vi "FPGA.vi"() -> ()   [LabVIEW 2013]
uses:
  <vilib>/rvi/Emulation/niFpgaSctlEmulationGetInTimedLoop.vi
  <vilib>/rvi/Emulation/niFpgaEmulationReportErrorSimple.vi
  <vilib>/rvi/eio/common/nirviEmuTemplateMethod_errors.vi
  <vilib>/rvi/Emulation/niFpgaGetClockAttributes.vi
  <vilib>/rvi/Emulation/niFpgaCriticalErrorInLSC.vi
  <vilib>/eio/EIONode/EIONode.xnode
panel:
  out "Test1":bool
  out "Test2":bool
  out "Test3":bool
  out "Test4":bool
  out "GbxEnc1":i64
  out "GbxEnc2":i64
  out "GbxEnc3":i64
  out "GbxEnc4":i64
  in  "FPGA LED":bool
  out "Chasis Temp":i16
  in  "Motor5":u16 max=512 step=1
  in  "Motor6":u16 max=512 step=1
  in  "Motor7":u16 max=512 step=1
  in  "Motor8":u16 max=512 step=1
  in  "Motor9":u16 max=512 step=1
  in  "Motor10":u16 max=512 step=1
  in  "Motor11":u16 max=512 step=1
  in  "Motor12":u16 max=512 step=1
  in  "Motor1":u16 max=512 step=1
  in  "Motor2":u16 max=512 step=1
  in  "Motor3":u16 max=512 step=1
  in  "Motor4":u16 max=512 step=1
  in  "Halt Execution":bool
  in  "Dout 1":bool
  in  "Dout 2":bool
  in  "Dout 3":bool
  in  "Dout 4":bool
  in  "Dout 5":bool
  in  "Dout 6":bool
  in  "Dout 7":bool
  in  "Dout 8":bool
  out "Din 1":bool
  out "Din 2":bool
  out "Din 3":bool
  out "Din 4":bool
  out "Din 5":bool
  out "Din 6":bool
  out "Din 7":bool
  out "Din 8":bool
  out "Encoder1":i64
  out "Encoder2":i64
  out "Encoder3":i64
  out "Encoder4":i64
  in  "Reset 1":bool
  in  "Reset 2":bool
  in  "Reset 3":bool
  in  "Reset 4":bool
  in  "Analog 2":fxp<+/-,12,5>
  in  "Analog 4":fxp<+/-,12,5>
  in  "Analog 1":fxp<+/-,12,5>
  in  "Analog 3":fxp<+/-,12,5>
  out "PWM counter":i16
  in  "Stop All Motors":bool
  in  "Status LED":bool
  in  "Emergency Stop":bool
  out "Enc1C":bool
  out "Enc2C":bool
  out "Enc3C":bool
  out "Enc4C":bool
  in  "Cal.1":bool
  in  "Cal.2":bool
  in  "Cal. 3":bool
  in  "Cal. 4":bool
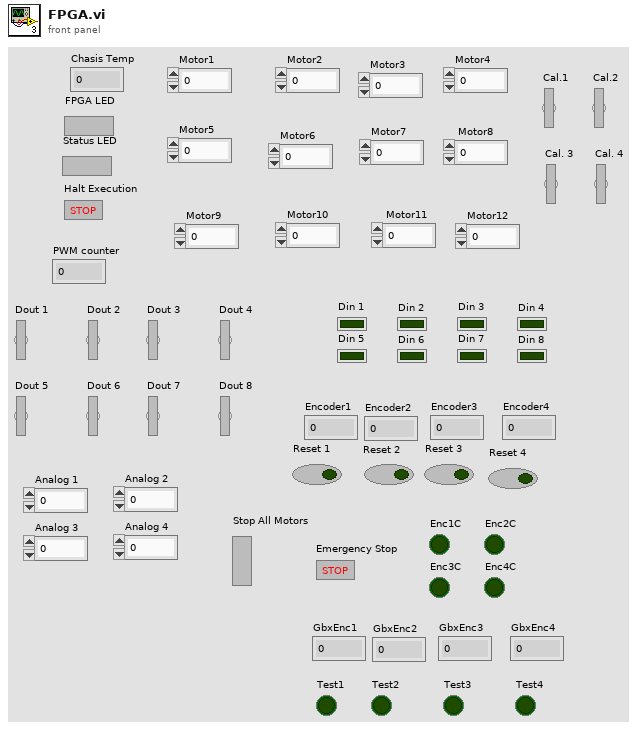
[diagram p1: front panel]
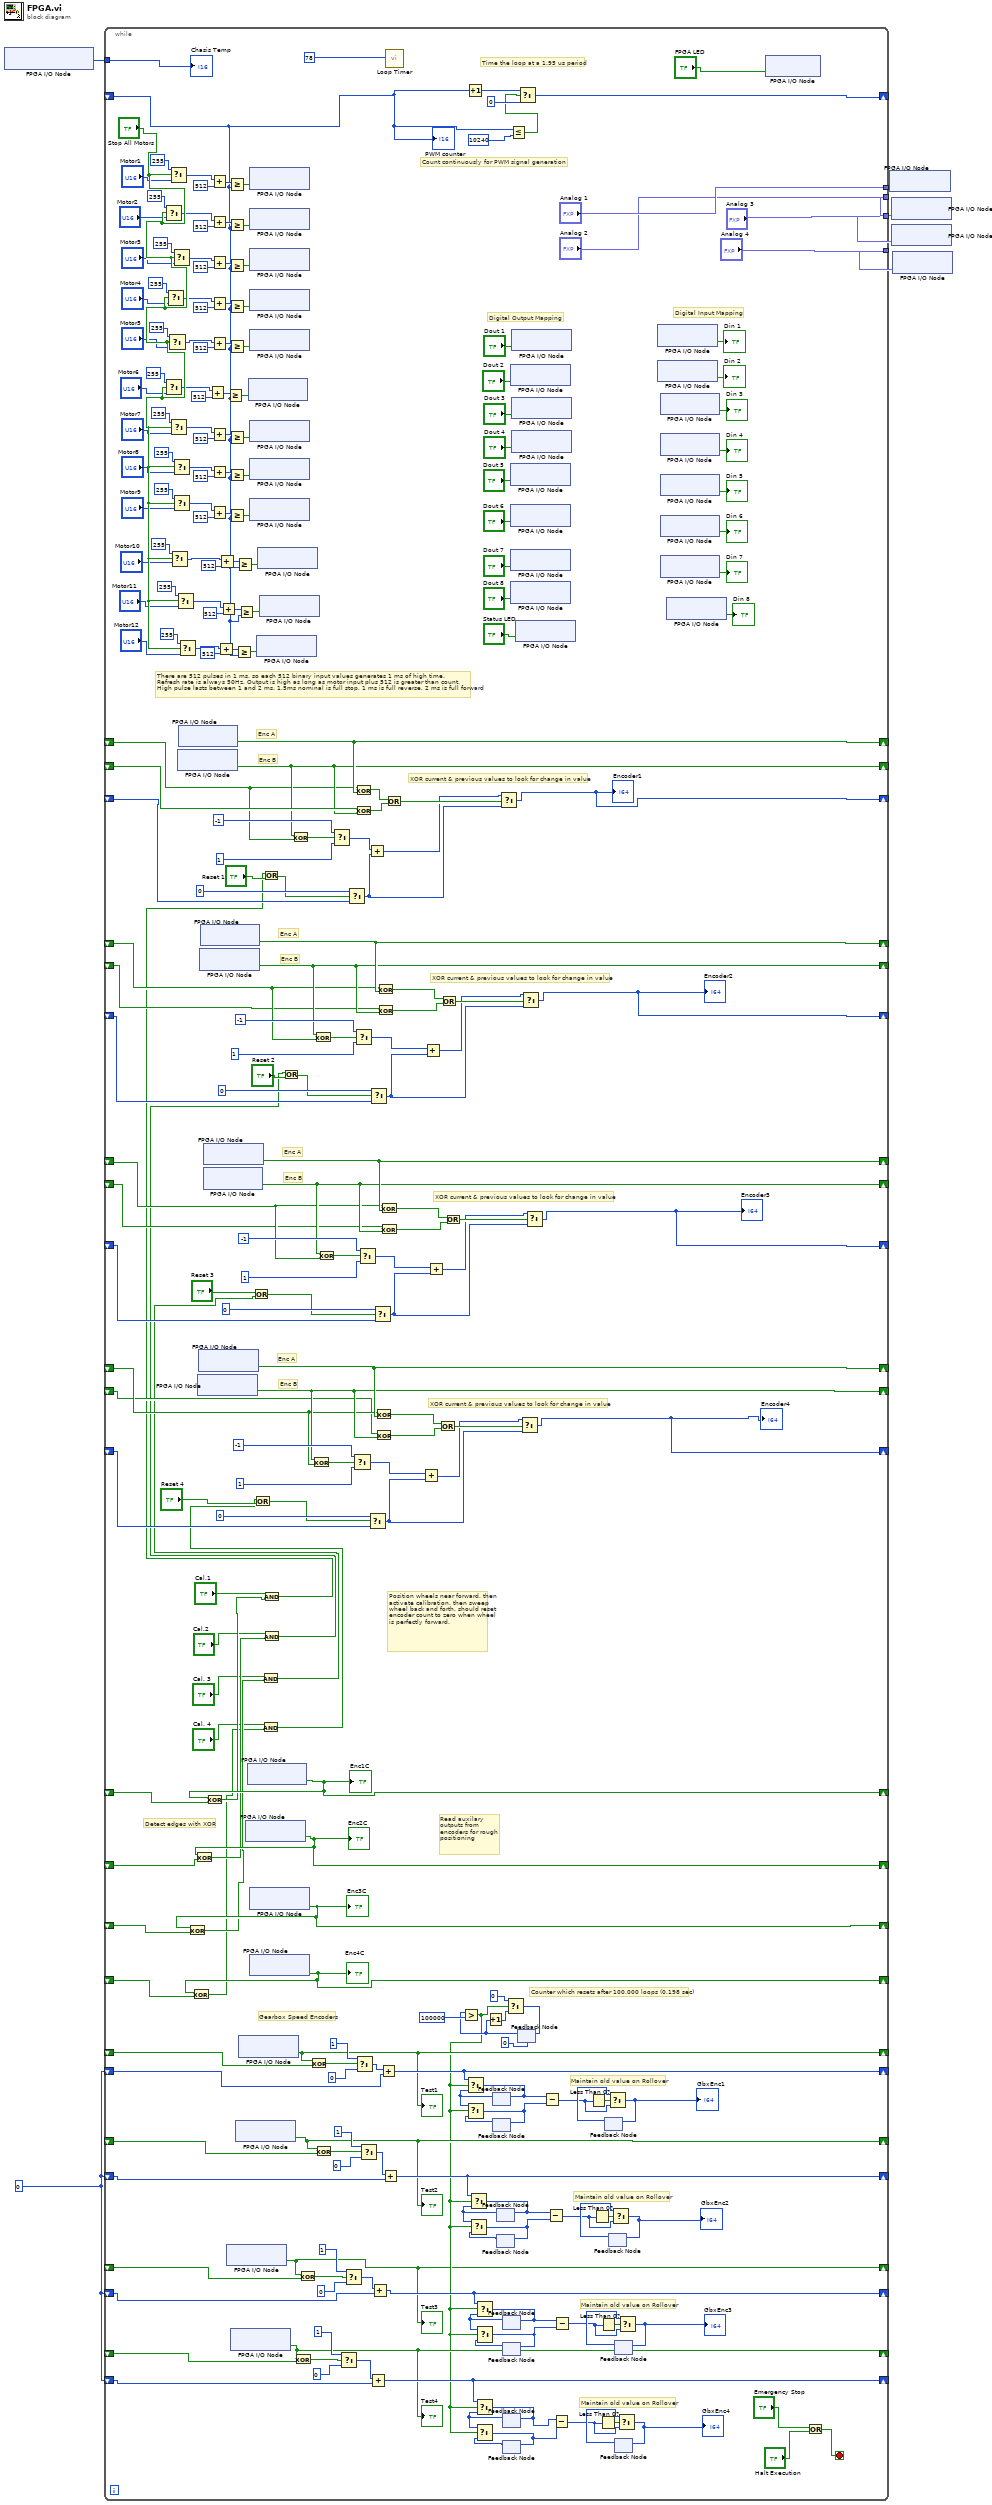
[diagram p0: block diagram]
diagram:
  w1 = u32 0
  n1 = xnode "FPGA I/O Node"() -> ("Chassis Temperature"=w6:i16)  [unwired: 1 in, 1 out]
  n2 = while {
    shift-right: [w223] -> _
    shift-left: _ -> [w207]
    shift-right: [w208] -> _
    shift-left: _ -> [w215]
    shift-right: [w217] -> _
    shift-left: _ -> [w216]
    shift-right: [w195] -> _
    shift-left: _ -> [w193]
    shift-right: [w194] -> _
    shift-left: _ -> [w192]
    shift-right: [w191] -> _
    shift-left: _ -> [w190]
    shift-right: [w179] -> _
    shift-left: _ -> [w177]
    shift-right: [w178] -> _
    shift-left: _ -> [w176]
    shift-right: [w174] -> _
    shift-left: _ -> [w175]
    shift-right: [w162] -> _
    shift-left: _ -> [w159]
    shift-right: [w161] -> _
    shift-left: _ -> [w158]
    shift-right: [w160] -> _
    shift-left: _ -> [w157]
    shift-right: [w152] -> _
    shift-left: _ -> [w151]
    tunnel: w6 -> [w149]
    tunnel: ["Analog 1"] -> w5
    tunnel: ["Analog 2"] -> w4
    tunnel: ["Analog 3"] -> w3
    tunnel: ["Analog 4"] -> w2
    shift-right: [w102] -> _
    shift-left: _ -> [w101]
    shift-right: [w100] -> _
    shift-left: _ -> [w99]
    shift-right: [w98] -> _
    shift-left: _ -> [w97]
    shift-right: [w95] -> _
    shift-left: _ -> [w96]
    shift-right: [w20] -> _
    shift-left: _ -> [w77]
    shift-right: [w19] -> _
    shift-left: _ -> [w64]
    shift-right: [w13] -> _
    shift-left: _ -> [w63]
    shift-right: [w17] -> _
    shift-left: _ -> [w62]
    shift-right: [w48] -> _
    shift-left: w1 -> [w57]
    shift-right: [w25] -> _
    shift-left: w1 -> [w56]
    shift-right: [w24] -> _
    shift-left: w1 -> [w55]
    shift-right: [w18] -> _
    shift-left: w1 -> [w54]
    stop <- w105 stop-if-true
    # "Maintain old value on Rollover"
    # "Maintain old value on Rollover"
    # "Maintain old value on Rollover"
    # "Maintain old value on Rollover"
    # "Counter which resets after 100,000 loops (0.198 sec)"
    # "Gearbox Speed Encoders"
    # "Position wheels near forward, then activate calibration, then sweep wheel back and forth. should reset encoder count to zero when wheel is perfectly forward."
    # "Detect edges with XOR"
    # "Read auxilary outputs from encoders for rough positioning"
    # "Count continuously for PWM signal generation"
    # "Time the loop at a 1.95 us period"
    # "XOR current & previous values to look for change in value"
    # "Enc B"
    # "Enc A"
    # "XOR current & previous values to look for change in value"
    # "Enc B"
    # "Enc A"
    # "XOR current & previous values to look for change in value"
    # "Enc B"
    # "Enc A"
    # "XOR current & previous values to look for change in value"
    # "Enc B"
    # "Enc A"
    # "Digital Input Mapping"
    # "Digital Output Mapping"
    # "There are 512 pulses in 1 ms, so each 512 binary input values generates 1 ms of high time.\nRefresh rate is always 50Hz. Output is high as long as motor input plus 512 is greater than count.\nHigh pulse lasts between 1 and 2 ms. 1.5ms nominal is full stop, 1 ms is full reverse, 2 ms is full forward"
    n3 = Select(t=i16 255, s="Stop All Motors", f="Motor2") -> (s? t:f=w128:u16)
    n4 = Select(t=i16 255, s="Stop All Motors", f="Motor6") -> (s? t:f=w120:u16)
    n5 = Select(t=i16 255, s="Stop All Motors", f="Motor4") -> (s? t:f=w124:u16)
    n6 = Select(t=i16 255, s="Stop All Motors", f="Motor5") -> (s? t:f=w122:u16)
    n7 = Select(t=i16 255, s="Stop All Motors", f="Motor1") -> (s? t:f=w130:u16)
    n8 = Select(t=i16 255, s="Stop All Motors", f="Motor7") -> (s? t:f=w118:u16)
    n9 = Select(t=i16 255, s="Stop All Motors", f="Motor10") -> (s? t:f=w112:u16)
    n10 = Select(t=i16 255, s="Stop All Motors", f="Motor3") -> (s? t:f=w126:u16)
    n11 = Select(t=i16 255, s="Stop All Motors", f="Motor8") -> (s? t:f=w116:u16)
    n12 = Select(t=i16 255, s="Stop All Motors", f="Motor9") -> (s? t:f=w114:u16)
    n13 = Select(t=i16 255, s="Stop All Motors", f="Motor11") -> (s? t:f=w110:u16)
    n14 = xnode "FPGA I/O Node"() -> ("Port7/DIO1"=w208:bool)  [unwired: 1 in, 1 out]
    n15 = xnode "FPGA I/O Node"() -> ("Port7/DIO0"=w223:bool)  [unwired: 1 in, 1 out]
    n16 = Select(t=i16 255, s="Stop All Motors", f="Motor12") -> (s? t:f=w108:u16)
    n17 = xnode "FPGA I/O Node"() -> ("Port4/DIO1"=w161:bool)  [unwired: 1 in, 1 out]
    n18 = xnode "FPGA I/O Node"() -> ("Port4/DIO0"=w162:bool)  [unwired: 1 in, 1 out]
    n19 = xnode "FPGA I/O Node"() -> ("Port3/DIO1"=w194:bool)  [unwired: 1 in, 1 out]
    n20 = xnode "FPGA I/O Node"() -> ("Port3/DIO0"=w195:bool)  [unwired: 1 in, 1 out]
    n21 = xnode "FPGA I/O Node"() -> ("Port3/DIO6"=w178:bool)  [unwired: 1 in, 1 out]
    n22 = xnode "FPGA I/O Node"() -> ("Port3/DIO5"=w179:bool)  [unwired: 1 in, 1 out]
    n23 = Add(x=w120, y=i16 512) -> (x+y=w265:u16)
    n24 = Add(x=w130, y=i16 512) -> (x+y=w275:u16)
    n25 = Add(x=w128, y=i16 512) -> (x+y=w273:u16)
    n26 = Add(x=w126, y=i16 512) -> (x+y=w271:u16)
    n27 = Add(x=w124, y=i16 512) -> (x+y=w269:u16)
    n28 = Add(x=w122, y=i16 512) -> (x+y=w267:u16)
    n29 = Add(x=w118, y=i16 512) -> (x+y=w263:u16)
    n30 = Add(x=w116, y=i16 512) -> (x+y=w261:u16)
    n31 = Add(x=w114, y=i16 512) -> (x+y=w259:u16)
    n32 = Add(x=w108, y=i16 512) -> (x+y=w253:u16)
    n33 = Add(x=w112, y=i16 512) -> (x+y=w257:u16)
    n34 = Add(x=w110, y=i16 512) -> (x+y=w255:u16)
    n35 = Greater Or Equal?(x=w265, y=w151) -> (x >= y?=w246:bool)
    n36 = xnode "FPGA I/O Node"() -> ("Port9/DIO2"=w13:bool)  [unwired: 1 in, 1 out]
    "Test3" <- w13
    n37 = Greater Or Equal?(x=w275, y=w151) -> (x >= y?=w251:bool)
    n38 = Greater Or Equal?(x=w273, y=w151) -> (x >= y?=w250:bool)
    n39 = Greater Or Equal?(x=w271, y=w151) -> (x >= y?=w249:bool)
    n40 = Greater Or Equal?(x=w269, y=w151) -> (x >= y?=w248:bool)
    n41 = Greater Or Equal?(x=w267, y=w151) -> (x >= y?=w247:bool)
    n42 = Greater Or Equal?(x=w263, y=w151) -> (x >= y?=w245:bool)
    n43 = Greater Or Equal?(x=w261, y=w151) -> (x >= y?=w244:bool)
    n44 = Greater Or Equal?(x=w259, y=w151) -> (x >= y?=w243:bool)
    n45 = xnode "FPGA I/O Node"() -> ("Port9/DIO9"=w17:bool)  [unwired: 1 in, 1 out]
    "Test4" <- w17
    n46 = Greater Or Equal?(x=w253, y=w151) -> (x >= y?=w240:bool)
    n47 = xnode "FPGA I/O Node"() -> ("Port9/DIO4"=w19:bool)  [unwired: 1 in, 1 out]
    "Test2" <- w19
    n48 = Greater Or Equal?(x=w257, y=w151) -> (x >= y?=w242:bool)
    n49 = Greater Or Equal?(x=w255, y=w151) -> (x >= y?=w241:bool)
    n50 = xnode "FPGA I/O Node"() -> ("Port9/DIO6"=w20:bool)  [unwired: 1 in, 1 out]
    "Test1" <- w20
    n51 = xnode "FPGA I/O Node"() -> ("Port3/DIO2"=w100:bool)  [unwired: 1 in, 1 out]
    "Enc2C" <- w100
    n52 = Exclusive Or(1:w99, 2:w100) -> (0:w93:bool)
    n53 = xnode "FPGA I/O Node"() -> ("Port7/DIO2"=w102:bool)  [unwired: 1 in, 1 out]
    "Enc1C" <- w102
    n54 = Exclusive Or(1:w101, 2:w102) -> (0:w94:bool)
    n55 = xnode "FPGA I/O Node"("Port0/DIO5"=w246) -> ()  [unwired: 1 in, 1 out]
    n56 = xnode "FPGA I/O Node"() -> ("Port4/DIO2"=w95:bool)  [unwired: 1 in, 1 out]
    "Enc4C" <- w95
    n57 = Exclusive Or(1:w96, 2:w95) -> (0:w91:bool)
    n58 = xnode "FPGA I/O Node"("Port0/DIO0"=w251) -> ()  [unwired: 1 in, 1 out]
    n59 = xnode "FPGA I/O Node"("Port0/DIO1"=w250) -> ()  [unwired: 1 in, 1 out]
    n60 = xnode "FPGA I/O Node"("Port0/DIO2"=w249) -> ()  [unwired: 1 in, 1 out]
    n61 = xnode "FPGA I/O Node"("Port0/DIO3"=w248) -> ()  [unwired: 1 in, 1 out]
    n62 = xnode "FPGA I/O Node"("Port0/DIO4"=w247) -> ()  [unwired: 1 in, 1 out]
    n63 = xnode "FPGA I/O Node"("Port0/DIO6"=w245) -> ()  [unwired: 1 in, 1 out]
    n64 = xnode "FPGA I/O Node"("Port0/DIO7"=w244) -> ()  [unwired: 1 in, 1 out]
    n65 = xnode "FPGA I/O Node"("Port0/DIO8"=w243) -> ()  [unwired: 1 in, 1 out]
    n66 = xnode "FPGA I/O Node"() -> ("Port3/DIO7"=w98:bool)  [unwired: 1 in, 1 out]
    "Enc3C" <- w98
    n67 = Exclusive Or(1:w97, 2:w98) -> (0:w92:bool)
    n68 = xnode "FPGA I/O Node"("Port1/DIO1"=w240) -> ()  [unwired: 1 in, 1 out]
    n69 = xnode "FPGA I/O Node"("Port1/DIO9"=w242) -> ()  [unwired: 1 in, 1 out]
    n70 = xnode "FPGA I/O Node"("Port1/DIO0"=w241) -> ()  [unwired: 1 in, 1 out]
    n71 = And(x="Cal. 3", y=w92) -> (x .and. y?=w79:bool)
    n72 = Or(x="Reset 3", y=w79) -> (x .or. y?=w84:bool)
    n73 = And(x="Cal. 4", y=w91) -> (x .and. y?=w78:bool)
    n74 = Or(x=w78, y="Reset 4") -> (x .or. y?=w85:bool)
    n75 = And(x="Cal.1", y=w94) -> (x .and. y?=w81:bool)
    n76 = Or(x=w81, y="Reset 1") -> (x .or. y?=w82:bool)
    n77 = And(x="Cal.2", y=w93) -> (x .and. y?=w80:bool)
    n78 = Or(x=w80, y="Reset 2") -> (x .or. y?=w83:bool)
    n79 = Exclusive Or(1:w207, 2:w208) -> (0:w209:bool)
    n80 = Exclusive Or(1:w62, 2:w17) -> (0:w65:bool)
    n81 = Exclusive Or(1:w63, 2:w13) -> (0:w68:bool)
    n82 = Exclusive Or(1:w77, 2:w20) -> (0:w74:bool)
    n83 = Exclusive Or(1:w159, 2:w161) -> (0:w163:bool)
    n84 = Exclusive Or(1:w193, 2:w194) -> (0:w197:bool)
    n85 = Exclusive Or(1:w64, 2:w19) -> (0:w71:bool)
    n86 = Exclusive Or(1:w177, 2:w178) -> (0:w180:bool)
    n87 = Select(t=i16 -1, s=w209, f=i16 1) -> (s? t:f=w211:i16)
    n88 = Select(t=i16 1, s=w65, f=i16 0) -> (s? t:f=w58:i16)
    n89 = Select(t=i16 1, s=w68, f=i16 0) -> (s? t:f=w59:i16)
    n90 = Select(t=i16 0, s=w82, f=w216) -> (s? t:f=w212:i16)
    n91 = Select(t=i16 -1, s=w163, f=i16 1) -> (s? t:f=w165:i16)
    n92 = Exclusive Or(1:w223, 2:w207) -> (0:w222:bool)
    n93 = Exclusive Or(1:w208, 2:w215) -> (0:w221:bool)
    n94 = Select(t=i16 -1, s=w197, f=i16 1) -> (s? t:f=w199:i16)
    n95 = Select(t=i16 1, s=w74, f=i16 0) -> (s? t:f=w61:i16)
    n96 = Select(t=i16 -1, s=w180, f=i16 1) -> (s? t:f=w182:i16)
    n97 = Select(t=i16 1, s=w71, f=i16 0) -> (s? t:f=w60:i16)
    n98 = Add(x=w211, y=w212) -> (x+y=w210:i16)
    n99 = Select(t=i16 0, s=w85, f=w157) -> (s? t:f=w166:i16)
    n100 = Add(x=w58, y=w54) -> (x+y=w18:u32)
    n101 = Select(t=i16 0, s=w83, f=w190) -> (s? t:f=w200:i16)
    n102 = Add(x=w59, y=w55) -> (x+y=w24:u32)
    n103 = Select(t=i16 0, s=w84, f=w175) -> (s? t:f=w183:i16)
    n104 = Exclusive Or(1:w162, 2:w159) -> (0:w172:bool)
    n105 = Exclusive Or(1:w161, 2:w158) -> (0:w171:bool)
    n106 = Exclusive Or(1:w195, 2:w193) -> (0:w206:bool)
    n107 = Exclusive Or(1:w194, 2:w192) -> (0:w205:bool)
    n108 = Add(x=w61, y=w57) -> (x+y=w48:u32)
    n109 = Exclusive Or(1:w179, 2:w177) -> (0:w189:bool)
    n110 = Exclusive Or(1:w178, 2:w176) -> (0:w188:bool)
    n111 = Add(x=w60, y=w56) -> (x+y=w25:u32)
    n112 = Or(x=w222, y=w221) -> (x .or. y?=w220:bool)
    n113 = call "Loop Timer"("Count(Ticks)"=i16 78) -> ()  [unwired: 1 out]
    n114 = Add(x=w165, y=w166) -> (x+y=w164:i16)
    n115 = Add(x=w199, y=w200) -> (x+y=w198:i16)
    n116 = Add(x=w182, y=w183) -> (x+y=w181:i16)
    n117 = Or(x=w172, y=w171) -> (x .or. y?=w170:bool)
    n118 = Or(x=w206, y=w205) -> (x .or. y?=w204:bool)
    n119 = Or(x=w189, y=w188) -> (x .or. y?=w187:bool)
    n120 = Increment(x=w151) -> (x+1=w156:i16)
    n121 = feedback #1() -> (w47:u32)  [unwired: 1 in]
    n122 = feedback #2() -> (w46:u32)  [unwired: 1 in]
    n123 = feedback #3() -> (w40:u32)  [unwired: 1 in]
    n124 = feedback #4() -> (w39:u32)  [unwired: 1 in]
    n125 = Select(t=w210, s=w220, f=w212) -> (s? t:f=w217:i16)
    "Encoder1" <- w217
    n126 = feedback #5() -> (w30:u32)  [unwired: 1 in]
    n127 = feedback #6() -> (w29:u32)  [unwired: 1 in]
    n128 = feedback #7() -> (w35:u32)  [unwired: 1 in]
    n129 = feedback #8() -> (w34:u32)  [unwired: 1 in]
    n130 = Less Or Equal?(x=w151, y=i16 10240) -> (x <= y?=w154:bool)
    n131 = xnode "FPGA I/O Node"("Port1/DIO3"="Dout 2") -> ()  [unwired: 1 in, 1 out]
    n132 = xnode "FPGA I/O Node"("Port1/DIO6"="Dout 5") -> ()  [unwired: 1 in, 1 out]
    n133 = xnode "FPGA I/O Node"("Port1/DIO7"="Dout 6") -> ()  [unwired: 1 in, 1 out]
    n134 = xnode "FPGA I/O Node"("Port1/DIO8"="Dout 7") -> ()  [unwired: 1 in, 1 out]
    n135 = xnode "FPGA I/O Node"("Port2/DIO9"="Dout 8") -> ()  [unwired: 1 in, 1 out]
    n136 = xnode "FPGA I/O Node"("Port1/DIO2"="Dout 1") -> ()  [unwired: 1 in, 1 out]
    n137 = xnode "FPGA I/O Node"("Port1/DIO4"="Dout 3") -> ()  [unwired: 1 in, 1 out]
    n138 = xnode "FPGA I/O Node"("Port1/DIO5"="Dout 4") -> ()  [unwired: 1 in, 1 out]
    n139 = xnode "FPGA I/O Node"("Port2/DIO1"="Status LED") -> ()  [unwired: 1 in, 1 out]
    n140 = feedback #9(u32 0) -> (w51:u32)
    n141 = Greater?(x=w51, y=u32 100000) -> (0:w16:bool)
    n142 = Select(t=w48, s=w16, f=w47) -> (s? t:f=w8:u32)
    n143 = Select(t=w47, s=w16, f=w46) -> (s? t:f=w7:u32)
    n144 = Select(t=w25, s=w16, f=w40) -> (s? t:f=w10:u32)
    n145 = Select(t=w40, s=w16, f=w39) -> (s? t:f=w9:u32)
    n146 = Select(t=w18, s=w16, f=w30) -> (s? t:f=w15:u32)
    n147 = Select(t=w30, s=w16, f=w29) -> (s? t:f=w14:u32)
    n148 = Select(t=w24, s=w16, f=w35) -> (s? t:f=w12:u32)
    n149 = Select(t=w35, s=w16, f=w34) -> (s? t:f=w11:u32)
    n150 = Increment(x=w51) -> (x+1=w52:u32)
    n151 = feedback-in #1(w8) -> ()
    n152 = feedback-in #2(w7) -> ()
    n153 = feedback-in #3(w10) -> ()
    n154 = feedback-in #4(w9) -> ()
    n155 = feedback-in #5(w15) -> ()
    n156 = feedback-in #6(w14) -> ()
    n157 = feedback-in #7(w12) -> ()
    n158 = feedback-in #8(w11) -> ()
    n159 = Select(t=u32 0, s=w16, f=w52) -> (s? t:f=w50:u32)
    n160 = feedback-in #9(w50) -> ()
    n161 = Select(t=w156, s=w154, f=i16 0) -> (s? t:f=w152:i16)
    n162 = Select(t=w164, s=w170, f=w166) -> (s? t:f=w160:i16)
    "Encoder4" <- w160
    n163 = Select(t=w198, s=w204, f=w200) -> (s? t:f=w191:i16)
    "Encoder2" <- w191
    n164 = Select(t=w181, s=w187, f=w183) -> (s? t:f=w174:i16)
    "Encoder3" <- w174
    n165 = Subtract(x=w8, y=w7) -> (x-y=w41:i64)
    n166 = Subtract(x=w10, y=w9) -> (x-y=w36:i64)
    n167 = Subtract(x=w15, y=w14) -> (x-y=w26:i64)
    n168 = Subtract(x=w12, y=w11) -> (x-y=w31:i64)
    n169 = Less Than 0?(x=w41) -> (x < 0?=w44:bool)
    n170 = Less Than 0?(x=w36) -> (x < 0?=w38:bool)
    n171 = Less Than 0?(x=w26) -> (x < 0?=w28:bool)
    n172 = Less Than 0?(x=w31) -> (x < 0?=w33:bool)
    n173 = feedback #10() -> (w42:i64)  [unwired: 1 in]
    n174 = Select(t=w42, s=w44, f=w41) -> (s? t:f=w43:i64)
    "GbxEnc1" <- w43
    n175 = feedback-in #10(w43) -> ()
    n176 = feedback #11() -> (w37:i64)  [unwired: 1 in]
    n177 = Select(t=w37, s=w38, f=w36) -> (s? t:f=w23:i64)
    "GbxEnc2" <- w23
    n178 = feedback-in #11(w23) -> ()
    n179 = feedback #12() -> (w27:i64)  [unwired: 1 in]
    n180 = feedback #13() -> (w32:i64)  [unwired: 1 in]
    n181 = Select(t=w27, s=w28, f=w26) -> (s? t:f=w21:i64)
    "GbxEnc4" <- w21
    n182 = feedback-in #12(w21) -> ()
    n183 = Select(t=w32, s=w33, f=w31) -> (s? t:f=w22:i64)
    "GbxEnc3" <- w22
    n184 = feedback-in #13(w22) -> ()
    n185 = xnode "FPGA I/O Node"() -> ("Port3/DIO8"=→"Din 1":bool)  [unwired: 1 in, 1 out]
    n186 = xnode "FPGA I/O Node"() -> ("Port4/DIO9"=→"Din 2":bool)  [unwired: 1 in, 1 out]
    n187 = xnode "FPGA I/O Node"() -> ("Port4/DIO3"=→"Din 3":bool)  [unwired: 1 in, 1 out]
    n188 = xnode "FPGA I/O Node"() -> ("Port4/DIO4"=→"Din 4":bool)  [unwired: 1 in, 1 out]
    n189 = xnode "FPGA I/O Node"() -> ("Port4/DIO5"=→"Din 5":bool)  [unwired: 1 in, 1 out]
    n190 = xnode "FPGA I/O Node"() -> ("Port4/DIO6"=→"Din 6":bool)  [unwired: 1 in, 1 out]
    n191 = xnode "FPGA I/O Node"() -> ("Port4/DIO7"=→"Din 7":bool)  [unwired: 1 in, 1 out]
    n192 = xnode "FPGA I/O Node"() -> ("Port4/DIO8"=→"Din 8":bool)  [unwired: 1 in, 1 out]
    n193 = xnode "FPGA I/O Node"("FPGA LED"="FPGA LED") -> ()  [unwired: 1 in, 1 out]
    n194 = Or(x="Emergency Stop", y="Halt Execution") -> (x .or. y?=w105:bool)
    "Chasis Temp" <- w149
    "PWM counter" <- w151
  }
  n195 = xnode "FPGA I/O Node"("ModB/AO0"=w5) -> ()  [unwired: 1 in, 1 out]
  n196 = xnode "FPGA I/O Node"("ModB/AO1"=w4) -> ()  [unwired: 1 in, 1 out]
  n197 = xnode "FPGA I/O Node"("ModB/AO2"=w3) -> ()  [unwired: 1 in, 1 out]
  n198 = xnode "FPGA I/O Node"("ModB/AO3"=w2) -> ()  [unwired: 1 in, 1 out]
